vi "Timer No Reset.vi"(9 "Direction":enum8{"either", "false-true", "true-false"}(ring), 10 "Tick Count(Ticks)":u32=40000000, 11 "Start Timer":bool) -> (3 "Timer Running":bool)   [LabVIEW 2020]
doc: "Author: Scott Hannahs <sth@magnet.fsu.edu>\nCopyright 2018 Florida State University, All rights reserved."
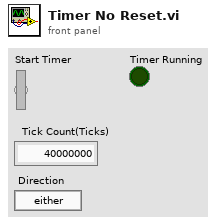
[diagram p1: front panel]
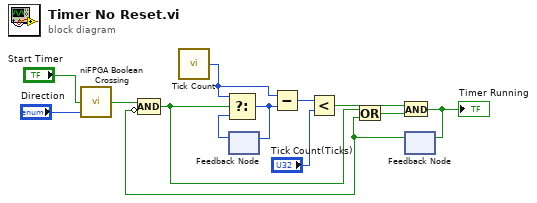
[diagram p0: block diagram]
diagram:
  n1 = call <vilib>:"niFPGA Boolean Crossing.vi"("input"="Start Timer", "direction"="Direction") -> ("crossing"=w3:bool)  [unwired: 7 in]
  n2 = call "Tick Count"() -> ("Tick Count(Ticks)"=w9:u32)
  n3 = feedback #1() -> (w11:u32)  [unwired: 1 in]
  n4 = feedback #2() -> (w1:bool)  [unwired: 1 in]
  n5 = Compound Arithmetic op=AND(w3, invert w1) -> (w2:bool)
  n6 = Select(t=w9, s=w2, f=w11) -> (s? t:f=w10:u32)
  n7 = feedback-in #1(w10) -> ()
  n8 = Subtract(x=w9, y=w10) -> (x-y=w8:u32)
  n9 = Less?(x=w8, y="Tick Count(Ticks)") -> (x < y?=w6:bool)
  n10 = Or(x=w2, y=w1) -> (x .or. y?=w4:bool)
  n11 = And(x=w6, y=w4) -> (x .and. y?=w5:bool)
  "Timer Running" <- w5
  n12 = feedback-in #2(w5) -> ()
